vi "Create Subpanel.vi"(5 "Scrollbars (off)":T2, 7 "Sizing":T1, 8 "error in (no error)":errorcluster, 9 "Subpanel Ref":refnum<vi>, 10 "UI VI Reference (caller)":refnum<vi>) -> (0 "error out":errorcluster, 3 "Flex Subpanel (Actor) out":refnum<class "Flex Subpanel (Actor).lvclass">)   [LabVIEW 2016, in "Flex UI Subpanel (Actor).lvlib" / "Flex Subpanel (Actor).lvclass"]
uses:
  Flex Subpanel (Actor).lvclass
  <vilib>/East West Architects/Flex UI/Flex UI Subpanel/Cluster - Scrollbar Visibility.ctl
  <vilib>/East West Architects/Flex UI/Flex UI Subpanel/Enum - Sizing.ctl
  <vilib>/East West Architects/Flex UI/Flex UI Subpanel/Flex UI Subpanel.lvclass
  C:/Program Files (x86)/National Instruments/LabVIEW 2016/vi.lib/East West Architects/Flex UI/Flex UI (Parent)/Flex UI.lvclass
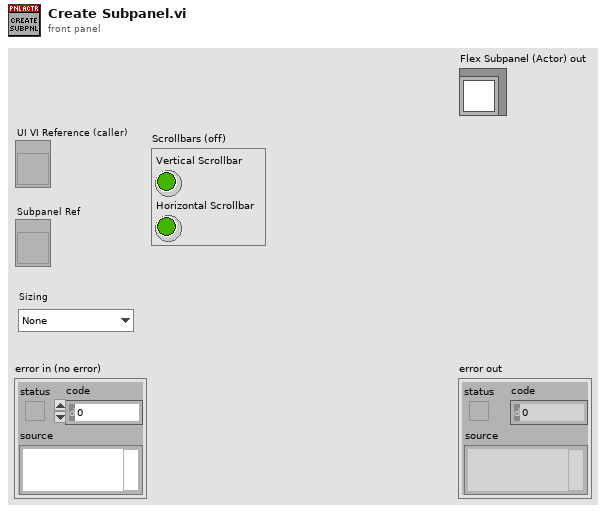
[diagram p1: front panel]
types:
  T1 = typedef "Flex UI Subpanel.lvclass/Enum - Sizing.ctl" = enum16{"None", "Largest Decoration", "Maximize"}
  T2 = typedef "Flex UI Subpanel.lvclass/Cluster - Scrollbar Visibility.ctl" = cluster{"Vertical Scrollbar":bool, "Horizontal Scrollbar":bool}
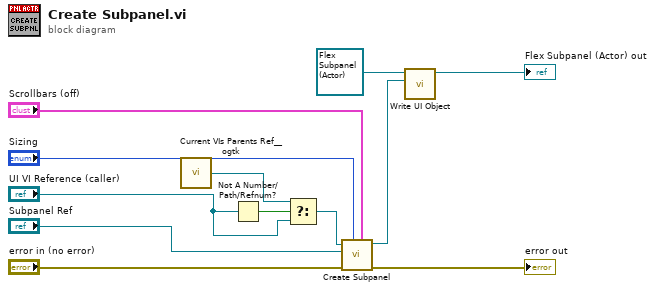
[diagram p0: block diagram]
diagram:
  n1 = call <userlib>:"Current VIs Parents Ref__ogtk.vi"() -> ("Calling VI's Reference"=w6:refnum<vi>)  [unwired: 2 in]
  n2 = Not A Number/Path/Refnum?(number/path/refnum="UI VI Reference (caller)") -> (NaN/Path/Refnum?=w7:bool)
  n3 = Select(t=w6, s=w7, f="UI VI Reference (caller)") -> (s? t:f=w5:refnum<vi>)
  n4 = call <vilib>:"Create Subpanel.vi"("Scrollbars (off)"="Scrollbars (off)", "Sizing"="Sizing", "error in"="error in (no error)", "Subpanel Ref"="Subpanel Ref", "UI VI Reference (caller)"=w5) -> ("error out"=→"error out":errorcluster, "Flex Subpanel out"=w8:refnum<class "Flex UI Subpanel.lvclass">)  [unwired: 5 in]
  n5 = call-dynamic "Write UI Object.vi"("Flex UI in"=w8, "Flex UI (Actor) in"=refnum<class "Flex Subpanel (Actor).lvclass"> refnum ("Flex UI Subpanel (Actor).lvlib:Flex Subpanel (Actor).lvclass")) -> ("Flex UI (Actor) out"=→"Flex Subpanel (Actor) out":refnum<class "Flex Subpanel (Actor).lvclass">)  [unwired: 8 in, 1 out]
